vi "Get Provided Interface.vi"(8 "error in (no error)":errorcluster, 11 "instrument in":refnum<class "Fake Instrument.lvclass">) -> (0 "error out":errorcluster, 2 "provided interface":string, 3 "instrument out":refnum<class "Fake Instrument.lvclass">)   [LabVIEW 2020, in "MeasurementServerTests.lvlib" / "Fake Instrument.lvclass"]
doc: "Returns the provided interface that will be used to query the MeasurmentLink Discovery Service for the address and port of the instrument's gRPC server. If your instrument does not use a gRPC server then you do not have to override this VI."
uses:
  Fake Instrument.lvclass
  Fake Instrument.lvclass/Fake Instrument.ctl
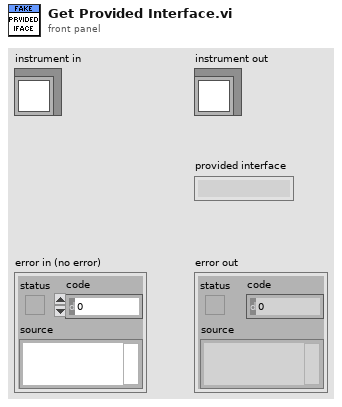
[diagram p1: front panel]
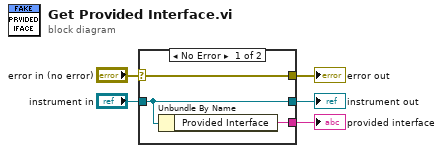
[diagram p0: block diagram]
diagram:
  n1 = case shown="No Error" "error in (no error)" {
    selector: "error in (no error)" -> [w8 w9]
    tunnel: "instrument in" -> [w7 w10]
    tunnel: [w7 w10] -> w4
    tunnel: [w8 w9] -> w2
    tunnel: [w6 _] -> w1
    frame No Error {
      n2 = Unbundle By Name(w7) -> ("Provided Interface"=w6:string)
    }
    frame Error {
    }
  }
  "error out" <- w2
  "instrument out" <- w4
  "provided interface" <- w1
